vi "InsertCRefLabelNode.vi"(6 "location":T2, 8 "error in (no error)":errorcluster, 9 "Type":T1, 10 "Name":string, 11 "Diagram":refnum<vi>) -> (0 "error out":errorcluster, 1 "Init Terminal":refnum<vi>, 2 "Ref Terminal":refnum<vi>, 3 "Diagram Out":refnum<vi>)   [LabVIEW 2012]
uses:
  <vilib>/Utility/miscctls.llb/LVPointTypeDef.ctl
  Core/Master Types.ctl
  CRef Label Node.xnode
  CRef.lvlib
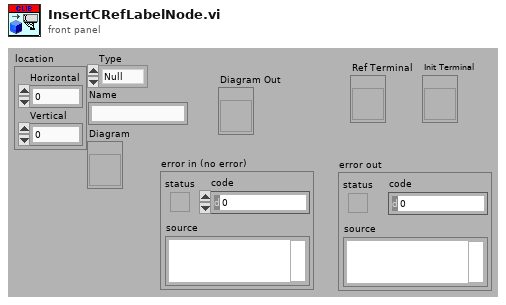
[diagram p1: front panel]
types:
  T1 = typedef "CRef.lvlib/Master Types.ctl" = enum8{"Null", "Boolean", "U8", "I8", "U16", "I16", "U32", "I32", "U64", "I64", "Single", "Double", "Extended", "CSG", "CDB", "CXT", "Boolean(Def)", "U8(Def)", "I8(Def)", "U16(Def)", "I16(Def)", "U32(Def)", "I32(Def)", "Reserved Def", "Reserved Def1", "Single(Def)", "Double(Def)", "Reserved Def2", "Reserved Def3", "Reserved Def4", "Reserved Def5", "Unsigned(Def)", "Signed(Def)", "Real(Def)", "Reserved Def6", "Numeric(Def)", "String"}
  T2 = typedef "LVPointTypeDef.ctl" = cluster{"Horizontal":i16, "Vertical":i16}
  T3 = cluster{"Library Version":cluster{"Major":u16, "Minor":u16, "Fix":u16, "Build":u16}, "State":variant}
  T4 = cluster{"Major":u16, "Minor":u16, "Fix":u16, "Build":u16}
  T5 = typedef "CRefScripting.lvlib/CRef Label Node.xnode/State.ctl" = cluster{"Name":string, "Hash":u32, "Type":T1}
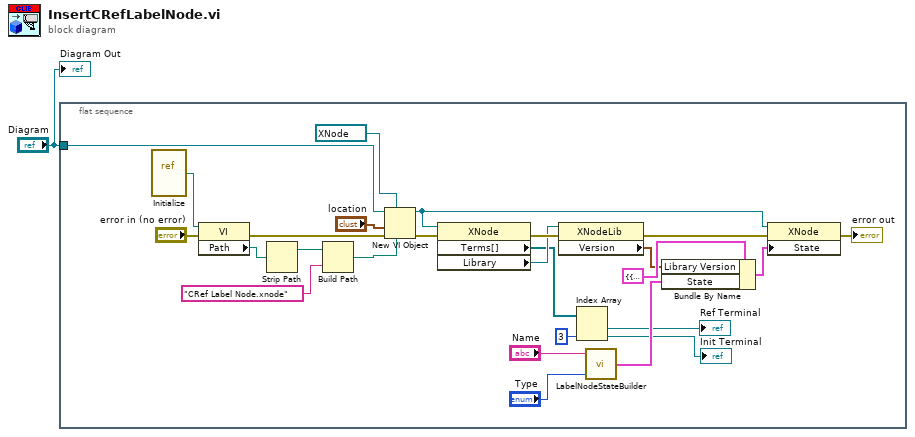
[diagram p0: block diagram]
diagram:
  n1 = flat-sequence {
    tunnel: "Diagram" -> [w27]
    frame #0 {
      n2 = vi-ref "Initialize.vi"() -> (w25:refnum<vi>)
      n3 = property class="VI"(reference=w25, error in="error in (no error)") -> (error out=w9:errorcluster, "Path"=w24:path)  [unwired: 1 out]
      n4 = Strip Path(path=w24) -> (stripped path=w23:path)  [unwired: 1 out]
      n5 = Build Path(base path=w23, name or relative path="CRef Label Node.xnode") -> (appended path=w22:path)
      n6 = New VI Object(vi object class=refnum<vi> refnum ("XRef"), owner refnum=w27, position/next to="location", 6:w22, 8:w9) -> (object refnum=w15:refnum<vi>, 0:w8:errorcluster)  [unwired: 3 in]
      n7 = property class="XNode"(reference=w15, error in=w8) -> (error out=w17:errorcluster, "Terms[]"=w5:refnum<vi>[], "Library"=w16:refnum<vi>)  [unwired: 1 out]
      n8 = property class="XNodeLib"(reference=w16, error in=w17) -> (error out=w13:errorcluster, "Version"=w14:T4)  [unwired: 1 out]
      n9 = Index Array(array=w5, index #2=3 ("index")) -> (element #1=→"Ref Terminal":refnum<vi>, element #2=→"Init Terminal":refnum<vi>)  [unwired: 1 in]
      n10 = call "LabelNodeStateBuilder.vi"("Reference Label"="Name", "Type"="Type") -> ("State Out"=w12:T5)  [unwired: 5 in, 2 out]
      n11 = Bundle By Name(cluster=T3 {"Library Version"={"Major"=0, "Minor"=0, "Fix"=0, "Build"=0}, "State"=variant} ("State"), "Library Version"=w14, "State"=w12) -> (w19:T3)
      n12 = property class="XNode"(reference=w15, error in=w13, "State"=w19) -> (error out=→"error out":errorcluster)  [unwired: 1 out]
    }
  }
  "Diagram Out" <- "Diagram"
